vi "战舰移动限制+导弹.vi"() -> ()   [LabVIEW 2018]
panel:
  out "数值":dbl
  out "战舰":T1
  out "激光武器1":T2
  out "激光武器 2":T2
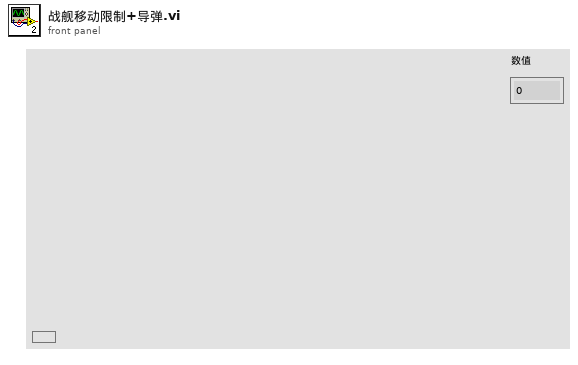
[diagram p1: front panel]
types:
  T1 = typedef "战列巡洋舰.ctl" = picture
  T2 = typedef "战列巡洋舰_激光武器.ctl" = picture
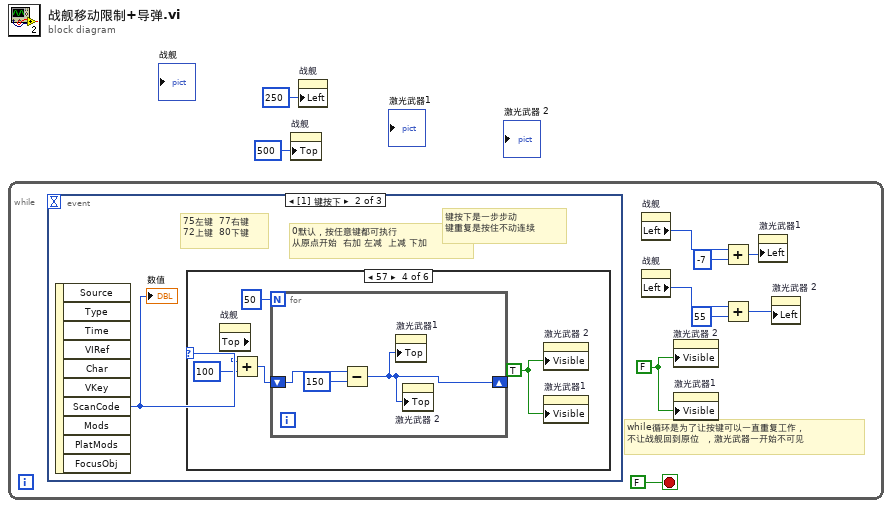
[diagram p0: block diagram]
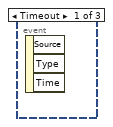
[diagram p2: hidden frame]
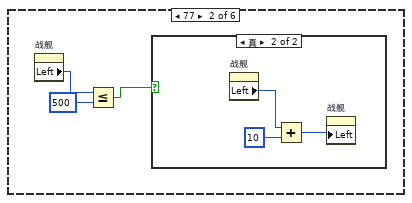
[diagram p4: hidden frame]
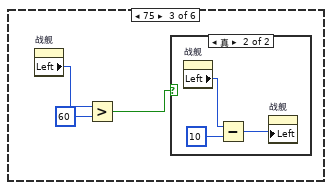
[diagram p6: hidden frame]
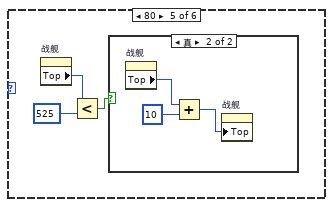
[diagram p8: hidden frame]
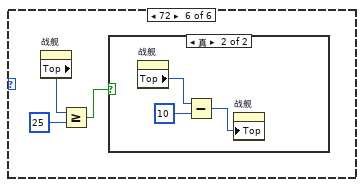
[diagram p10: hidden frame]
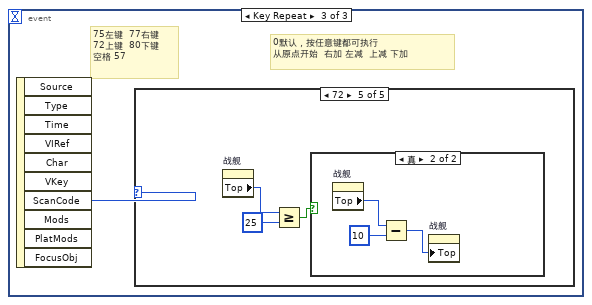
[diagram p12: hidden frame]
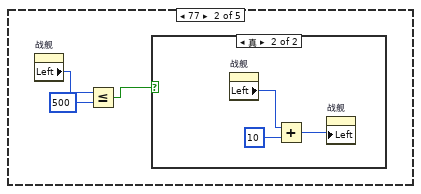
[diagram p14: hidden frame]
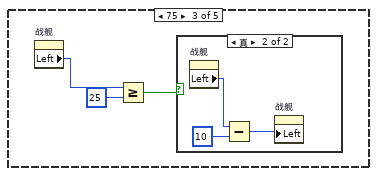
[diagram p16: hidden frame]
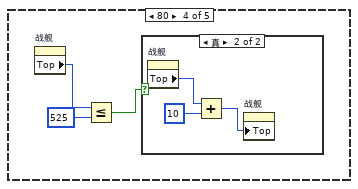
[diagram p18: hidden frame]
diagram:
  n1 = while {
    stop <- FALSE stop-if-true
    w3 = FALSE
    # "while循环是为了让按键可以一直重复工作，\n不让战舰回到原位  ，激光武器一开始不可见"
    n2 = event shown="[1] 键按下" {
      selector: _ -> [_ _ _]
      dyn-events: _ -> [_ _ _]
      timeout: _ -> [_ _ _]
      event Timeout {
        n3 = event-data() -> ()  [unwired: 1 in, 3 out]
      }
      event Key Down {
        # "键按下是一步步动\n键重复是按住不动连续"
        # "75左键  77右键\n72上键  80下键"
        # "0默认，按任意键都可执行\n从原点开始  右加 左减  上减 下加"
        n4 = event-data() -> ("ScanCode"=w11:i16)  [unwired: 1 in, 9 out]
        "数值" <- w11
        n5 = case shown="57" w11 {
          frame 0, Default {
          }
          frame 77 {
            n6 = property on="战舰" class="Pict (严格)"() -> ("Left"=w14:i32)  [unwired: 2 in, 2 out]
            n7 = Less Or Equal?(x=w14, y=500) -> (x <= y?=w12:bool)
            n8 = case shown="真" w12 {
              frame False {
              }
              frame True {
                n9 = property on="战舰" class="Pict (严格)"() -> ("Left"=w16:i32)  [unwired: 2 in, 2 out]
                n10 = Add(x=w16, y=10) -> (x+y=w17:i32)
                n11 = property on="战舰" class="Pict (严格)"("Left"=w17) -> ()  [unwired: 2 in, 2 out]
              }
            }
          }
          frame 75 {
            n12 = property on="战舰" class="Pict (严格)"() -> ("Left"=w20:i32)  [unwired: 2 in, 2 out]
            n13 = Greater?(x=w20, y=60) -> (0:w18:bool)
            n14 = case shown="真" w18 {
              frame False {
              }
              frame True {
                n15 = property on="战舰" class="Pict (严格)"() -> ("Left"=w22:i32)  [unwired: 2 in, 2 out]
                n16 = Subtract(x=w22, y=10) -> (x-y=w23:i32)
                n17 = property on="战舰" class="Pict (严格)"("Left"=w23) -> ()  [unwired: 2 in, 2 out]
              }
            }
          }
          frame 57 {
            w24 = TRUE
            n18 = property on="战舰" class="Pict (严格)"() -> ("Top"=w27:i32)  [unwired: 2 in, 2 out]
            n19 = Add(x=w27, y=100) -> (x+y=w25:i32)
            n20 = for {
              N: 50 -> [_]
              shift-right: [w29] -> _
              shift-left: w25 -> [w31]
              n21 = Subtract(x=w31, y=150) -> (x-y=w29:i32)
              n22 = property on="激光武器1" class="Pict (严格)"("Top"=w29) -> ()  [unwired: 2 in, 2 out]
              n23 = property on="激光武器 2" class="Pict (严格)"("Top"=w29) -> ()  [unwired: 2 in, 2 out]
            }
            n24 = property on="激光武器 2" class="Pict (严格)"("Visible"=w24) -> ()  [unwired: 2 in, 2 out]
            n25 = property on="激光武器1" class="Pict (严格)"("Visible"=w24) -> ()  [unwired: 2 in, 2 out]
          }
          frame 80 {
            n26 = property on="战舰" class="Pict (严格)"() -> ("Top"=w34:i32)  [unwired: 2 in, 2 out]
            n27 = Less?(x=w34, y=525) -> (x < y?=w32:bool)
            n28 = case shown="真" w32 {
              frame False {
              }
              frame True {
                n29 = property on="战舰" class="Pict (严格)"() -> ("Top"=w36:i32)  [unwired: 2 in, 2 out]
                n30 = Add(x=w36, y=10) -> (x+y=w35:i32)
                n31 = property on="战舰" class="Pict (严格)"("Top"=w35) -> ()  [unwired: 2 in, 2 out]
              }
            }
          }
          frame 72 {
            n32 = property on="战舰" class="Pict (严格)"() -> ("Top"=w40:i32)  [unwired: 2 in, 2 out]
            n33 = Greater Or Equal?(x=w40, y=25) -> (x >= y?=w39:bool)
            n34 = case shown="真" w39 {
              frame False {
              }
              frame True {
                n35 = property on="战舰" class="Pict (严格)"() -> ("Top"=w43:i32)  [unwired: 2 in, 2 out]
                n36 = Subtract(x=w43, y=10) -> (x-y=w42:i32)
                n37 = property on="战舰" class="Pict (严格)"("Top"=w42) -> ()  [unwired: 2 in, 2 out]
              }
            }
          }
        }
      }
      event Key Repeat {
        # "75左键  77右键\n72上键  80下键\n空格 57"
        # "0默认，按任意键都可执行\n从原点开始  右加 左减  上减 下加"
        n38 = event-data() -> ("ScanCode"=w44:i16)  [unwired: 1 in, 9 out]
        n39 = case shown="72" w44 {
          frame 0, Default {
          }
          frame 77 {
            n40 = property on="战舰" class="Pict (严格)"() -> ("Left"=w47:i32)  [unwired: 2 in, 2 out]
            n41 = Less Or Equal?(x=w47, y=500) -> (x <= y?=w46:bool)
            n42 = case shown="真" w46 {
              frame False {
              }
              frame True {
                n43 = property on="战舰" class="Pict (严格)"() -> ("Left"=w49:i32)  [unwired: 2 in, 2 out]
                n44 = Add(x=w49, y=10) -> (x+y=w50:i32)
                n45 = property on="战舰" class="Pict (严格)"("Left"=w50) -> ()  [unwired: 2 in, 2 out]
              }
            }
          }
          frame 75 {
            n46 = property on="战舰" class="Pict (严格)"() -> ("Left"=w53:i32)  [unwired: 2 in, 2 out]
            n47 = Greater Or Equal?(x=w53, y=25) -> (x >= y?=w52:bool)
            n48 = case shown="真" w52 {
              frame False {
              }
              frame True {
                n49 = property on="战舰" class="Pict (严格)"() -> ("Left"=w56:i32)  [unwired: 2 in, 2 out]
                n50 = Subtract(x=w56, y=10) -> (x-y=w55:i32)
                n51 = property on="战舰" class="Pict (严格)"("Left"=w55) -> ()  [unwired: 2 in, 2 out]
              }
            }
          }
          frame 80 {
            n52 = property on="战舰" class="Pict (严格)"() -> ("Top"=w59:i32)  [unwired: 2 in, 2 out]
            n53 = Less Or Equal?(x=w59, y=525) -> (x <= y?=w58:bool)
            n54 = case shown="真" w58 {
              frame False {
              }
              frame True {
                n55 = property on="战舰" class="Pict (严格)"() -> ("Top"=w61:i32)  [unwired: 2 in, 2 out]
                n56 = Add(x=w61, y=10) -> (x+y=w60:i32)
                n57 = property on="战舰" class="Pict (严格)"("Top"=w60) -> ()  [unwired: 2 in, 2 out]
              }
            }
          }
          frame 72 {
            n58 = property on="战舰" class="Pict (严格)"() -> ("Top"=w65:i32)  [unwired: 2 in, 2 out]
            n59 = Greater Or Equal?(x=w65, y=25) -> (x >= y?=w64:bool)
            n60 = case shown="真" w64 {
              frame False {
              }
              frame True {
                n61 = property on="战舰" class="Pict (严格)"() -> ("Top"=w68:i32)  [unwired: 2 in, 2 out]
                n62 = Subtract(x=w68, y=10) -> (x-y=w67:i32)
                n63 = property on="战舰" class="Pict (严格)"("Top"=w67) -> ()  [unwired: 2 in, 2 out]
              }
            }
          }
        }
      }
    }
    n64 = property on="战舰" class="Pict (严格)"() -> ("Left"=w9:i32)  [unwired: 2 in, 2 out]
    n65 = property on="战舰" class="Pict (严格)"() -> ("Left"=w5:i32)  [unwired: 2 in, 2 out]
    n66 = property on="激光武器 2" class="Pict (严格)"("Visible"=w3) -> ()  [unwired: 2 in, 2 out]
    n67 = property on="激光武器1" class="Pict (严格)"("Visible"=w3) -> ()  [unwired: 2 in, 2 out]
    n68 = Add(x=w9, y=-7) -> (x+y=w8:i32)
    n69 = Add(x=w5, y=55) -> (x+y=w4:i32)
    n70 = property on="激光武器1" class="Pict (严格)"("Left"=w8) -> ()  [unwired: 2 in, 2 out]
    n71 = property on="激光武器 2" class="Pict (严格)"("Left"=w4) -> ()  [unwired: 2 in, 2 out]
  }
  n72 = property on="战舰" class="Pict (严格)"("Top"=500 ("位置:置顶")) -> ()  [unwired: 2 in, 2 out]
  n73 = property on="战舰" class="Pict (严格)"("Left"=250 ("位置:居左")) -> ()  [unwired: 2 in, 2 out]
